vi "GetFreqOffset_Addon.vi"(8 "Error In":errorcluster, 9 "Resp Timeout (ms)":i32 min=0, 10 "Enum":T1, 11 "FPGA Reference":refnum<k20>) -> (0 "Error Out":errorcluster, 1 "Freq Offset (Hz)":ext, 2 "Get Freq Offset OK":bool, 3 "Received Text":string)   [LabVIEW 2018]
uses:
  Resources_Test/UART/ControlTestSlot.ctl
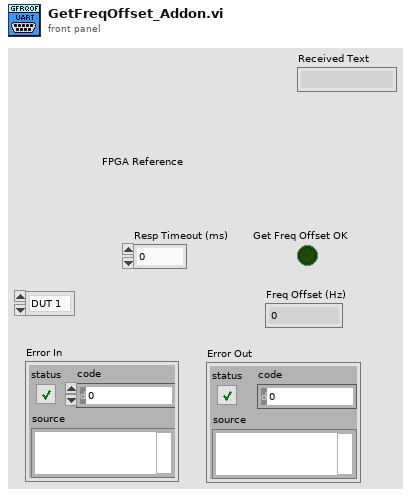
[diagram p1: front panel]
types:
  T1 = typedef "ControlTestSlot.ctl" = enum16{"DUT 1", "DUT 2"}
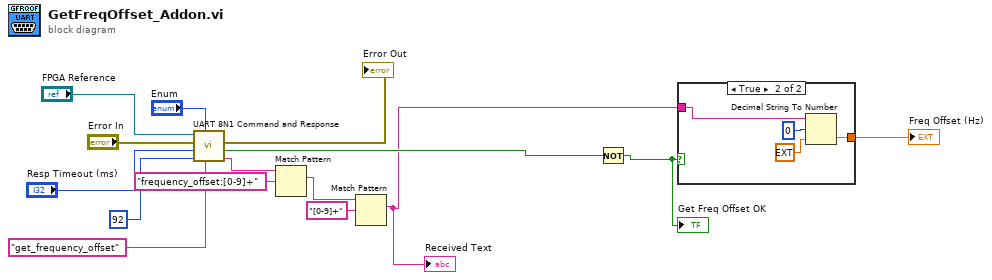
[diagram p0: block diagram]
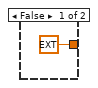
[diagram p2: hidden frame]
diagram:
  n1 = call "UART 8N1 Command and Response.vi"("Text to Send"="get_frequency_offset", "Active Dut"="Enum", "Response Size (char)"=u32 92, "Response Timeout (ms)"="Resp Timeout (ms)", "Error In"="Error In", "FPGA VI Reference In"="FPGA Reference") -> ("Received Text"=w7:string, "Timeout Flag"=w8:bool, "Error Out"=→"Error Out":errorcluster)  [unwired: 1 in, 2 out]
  n2 = Match Pattern(string=w7, regular expression="frequency_offset:[0-9]+") -> (match substring=w5:string)  [unwired: 1 in, 3 out]
  n3 = Match Pattern(string=w5, regular expression="[0-9]+") -> (match substring=w2:string)  [unwired: 1 in, 3 out]
  "Received Text" <- w2
  n4 = Not(x=w8) -> (.not. x?=w3:bool)
  "Get Freq Offset OK" <- w3
  n5 = case shown="True" w3 {
    tunnel: w2 -> [_ w17]
    tunnel: [ext 0.0 w18] -> w1
    frame False {
    }
    frame True {
      n6 = Decimal String To Number(string=w17, offset=0, default (0L)=ext 0.0 ("default (0 I32)")) -> (number=w18:ext)  [unwired: 1 out]
    }
  }
  "Freq Offset (Hz)" <- w1
